vi "Test_AddMultipleToList_RetrieveList.vi"(8 "error in (no error)":errorcluster, 11 "TestCase in":refnum<class "TestStringList.lvclass">) -> (0 "error out":errorcluster, 3 "TestCase out":refnum<class "TestStringList.lvclass">)   [LabVIEW 2015, in "StringList.lvlib" / "TestStringList.lvclass"]
uses:
  TestStringList.lvclass
  <vilib>/addons/_JKI Toolkits/VI Tester/TestCase.llb/TestCase.lvclass
  StringList.lvclass
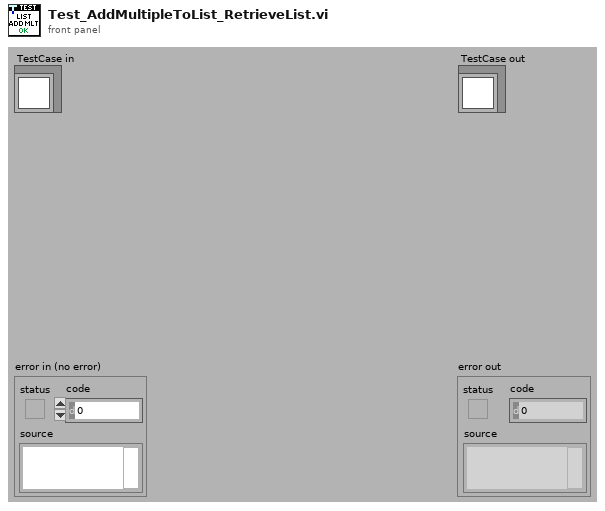
[diagram p1: front panel]
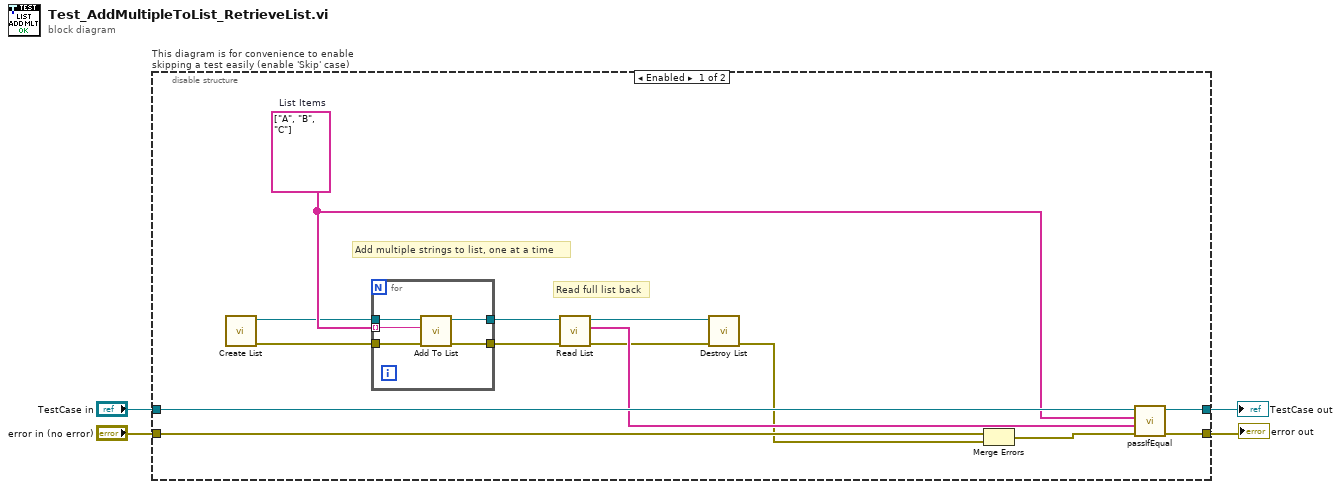
[diagram p0: block diagram]
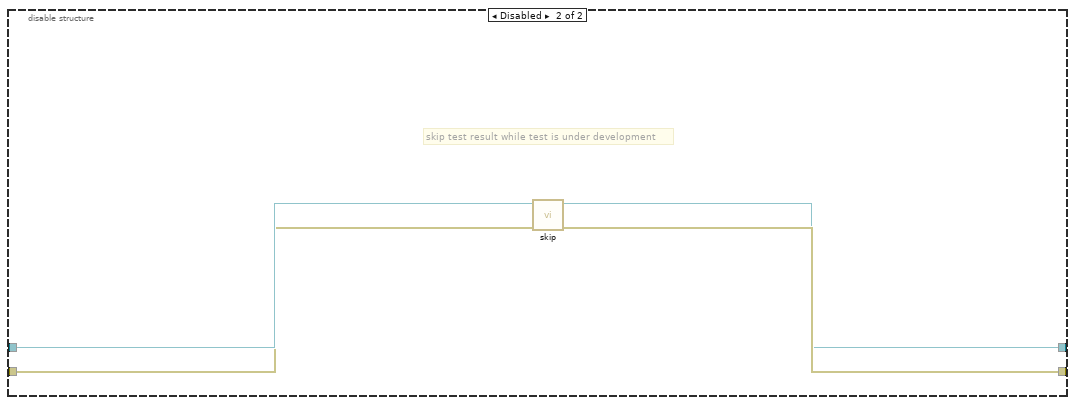
[diagram p2: hidden frame]
diagram:
  n1 = disable-structure "This diagram is for convenience to enable skipping a test easily (enable 'Skip' case)" shown="Enabled" {
    disable-tunnel: "TestCase in" -> [w18 w27]
    disable-tunnel: [w17 w25] -> w1
    disable-tunnel: [w16 w26] -> w3
    disable-tunnel: "error in (no error)" -> [w15 w24]
    frame Enabled {
      w12 = string[] ["A", "B", "C"]  # List Items
      # "Read full list back"
      # "Add multiple strings to list, one at a time"
      n2 = call "Create List.vi"() -> ("error out"=w8:errorcluster, "StringList Reference"=w11:refnum<data-value>)  [unwired: 10 in]
      n3 = for {
        tunnel: w12 -> [w21] mode=indexing
        tunnel: w11 -> [w23]
        tunnel: [w22] -> w13
        tunnel: w8 -> [w20]
        tunnel: [w19] -> w7
        n4 = call "Add To List.vi"("error in (no error)"=w20, "Item"=w21, "StringList Reference"=w23) -> ("error out"=w19:errorcluster, "StringList Reference"=w22:refnum<data-value>)  [unwired: 7 in]
      }
      n5 = call "Read List.vi"("error in (no error)"=w7, "StringList Reference"=w13) -> ("error out"=w6:errorcluster, "Items"=w14:string[], "StringList Reference"=w9:refnum<data-value>)  [unwired: 7 in]
      n6 = call "Destroy List.vi"("error in (no error)"=w6, "StringList Reference"=w9) -> ("error out"=w5:errorcluster)  [unwired: 8 in, 1 out]
      n7 = Merge Errors(w15, w5) -> (w10:errorcluster)
      n8 = call-dynamic "passIfEqual.vi"("error in (no error)"=w10, "y"=w14, "x"=w12, "TestCase in"=w18) -> ("error out"=w16:errorcluster, "TestCase out"=w17:refnum<class "TestStringList.lvclass">)  [unwired: 6 in]
    }
    frame Disabled {
      # "skip test result while test is under development"
      n9 = call <vilib>:"skip.vi"("error in (no error)"=w24, "TestCase in"=w27) -> ("error out"=w26:errorcluster, "TestCase out"=w25:refnum<class "TestStringList.lvclass">)  [unwired: 8 in]
    }
  }
  "error out" <- w3
  "TestCase out" <- w1
